vi "VITester_Provider_InitItems.vi"(11 "Items Array":T1[](array[typedef])) -> ()   [LabVIEW 2013]
uses:
  Support/VITester Project Item Ref.ctl
panel:
  out "error out":errorcluster
  in  "error in":errorcluster
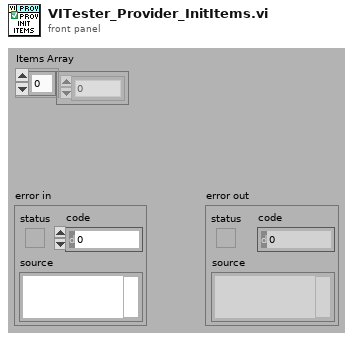
[diagram p1: front panel]
types:
  T1 = typedef "VITester Project Item Ref.ctl" = u64
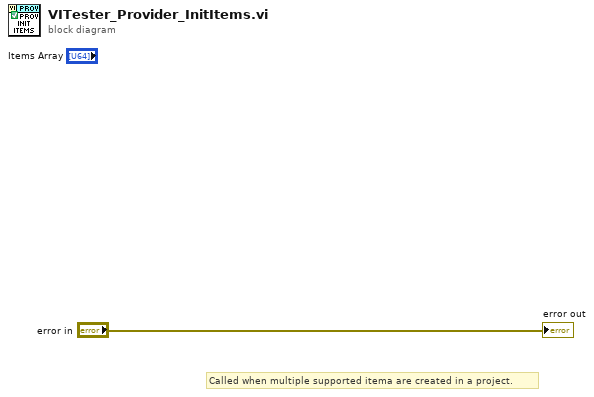
[diagram p0: block diagram]
diagram:
  # "Called when multiple supported itema are created in a project."
  "error out" <- "error in"
